vi "Top Level.vi"() -> ()   [LabVIEW 2020]
uses:
  Users/josferna/OneDrive - NI/Documents/Accounts&Proojects/Open Case Files/01072359 - Microsoft/rad-master/subVIs/rad_Globals.vi
  Users/josferna/OneDrive - NI/Documents/Accounts&Proojects/Open Case Files/01072359 - Microsoft/rad-master/subVIs/Util/Controls/Exit Button.ctl
  Users/josferna/OneDrive - NI/Documents/Accounts&Proojects/Open Case Files/01072359 - Microsoft/rad-master/subVIs/Util/FP Control/FP Control Functions.ctl
  <vilib>/Utility/miscctls.llb/LVRowAndColumnUnsignedTypeDef.ctl
  <vilib>/nisyscfg/nisyscfg.lvlib
  <resource>/objmgr/nisysapi.rc
  Users/josferna/OneDrive - NI/Documents/Accounts&Proojects/Open Case Files/01072359 - Microsoft/rad-master/subVIs/RT Image Compare/TypeDefs/rad_Comparison Modes.ctl
  Users/josferna/OneDrive - NI/Documents/Accounts&Proojects/Open Case Files/01072359 - Microsoft/rad-master/subVIs/Targets/TypeDefs/rad_Target Network Settings.ctl
  Users/josferna/OneDrive - NI/Documents/Accounts&Proojects/Open Case Files/01072359 - Microsoft/rad-master/subVIs/Targets/TypeDefs/rad_Target Information.ctl
  <vilib>/nisyscfg/Close (System).vi
  Users/josferna/OneDrive - NI/Documents/Accounts&Proojects/Open Case Files/01072359 - Microsoft/rad-master/subVIs/Util/Controls/Refresh Button.ctl
  Users/josferna/OneDrive - NI/Documents/Accounts&Proojects/Open Case Files/01072359 - Microsoft/rad-master/subVIs/Util/Controls/Add Target Button.ctl
  Users/josferna/OneDrive - NI/Documents/Accounts&Proojects/Open Case Files/01072359 - Microsoft/rad-master/subVIs/Util/Controls/Configure Button.ctl
  Users/josferna/OneDrive - NI/Documents/Accounts&Proojects/Open Case Files/01072359 - Microsoft/rad-master/subVIs/Util/Controls/Select All Button.ctl
  Users/josferna/OneDrive - NI/Documents/Accounts&Proojects/Open Case Files/01072359 - Microsoft/rad-master/subVIs/Util/Controls/Compare Button.ctl
  Users/josferna/OneDrive - NI/Documents/Accounts&Proojects/Open Case Files/01072359 - Microsoft/rad-master/subVIs/Util/Controls/Retrieve Button.ctl
  Users/josferna/OneDrive - NI/Documents/Accounts&Proojects/Open Case Files/01072359 - Microsoft/rad-master/subVIs/Util/Controls/Deploy Button.ctl
  Users/josferna/OneDrive - NI/Documents/Accounts&Proojects/Open Case Files/01072359 - Microsoft/rad-master/subVIs/App Images/TypeDefs/rad_FPGA Flash Properties.ctl
  Users/josferna/OneDrive - NI/Documents/Accounts&Proojects/Open Case Files/01072359 - Microsoft/rad-master/subVIs/App Images/TypeDefs/rad_FPGA Properties.ctl
  Users/josferna/OneDrive - NI/Documents/Accounts&Proojects/Open Case Files/01072359 - Microsoft/rad-master/subVIs/App Images/TypeDefs/rad_Application Image Properties.ctl
  Users/josferna/OneDrive - NI/Documents/Accounts&Proojects/Open Case Files/01072359 - Microsoft/rad-master/subVIs/App Images/TypeDefs/rad_AppImage Information.ctl
  Users/josferna/OneDrive - NI/Documents/Accounts&Proojects/Open Case Files/01072359 - Microsoft/rad-master/subVIs/App Images/TypeDefs/rad_App Images Settings.ctl
  Users/josferna/OneDrive - NI/Documents/Accounts&Proojects/Open Case Files/01072359 - Microsoft/rad-master/subVIs/Targets/TypeDefs/rad_Targets Settings.ctl
  Users/josferna/OneDrive - NI/Documents/Accounts&Proojects/Open Case Files/01072359 - Microsoft/rad-master/subVIs/Targets/TypeDefs/rad_Discovery Settings.ctl
  Users/josferna/OneDrive - NI/Documents/Accounts&Proojects/Open Case Files/01072359 - Microsoft/rad-master/subVIs/TypeDefs/rad_State Data.ctl
panel:
  in  "App Images List 2":i32(listbox)=6
  in  "Target List 2":i32[](listbox)=[0]
  in  "State":T1 {"Targets Information"."Primary NIC"."IP Address Request Mode" items=["Static"=1, "DHCP/Link-Local"=2, "Link-Local Only"=4, "DHCP Only"=8]}
  in  "Exit":T11
  in  "Deploy":T12
  in  "Retrieve":T13
  in  "Compare":T14
  in  "Configure App":T15
  in  "Select All":T16
  in  "Configure Targets":T15
  in  "App Images Settings":bool
  in  "Add Target":T17
  in  "Targets Settings":bool
  in  "Refresh Apps":T18
  in  "App Images List":i32(listbox)=6
  in  "Target List":i32[](listbox)=[0]
  in  "Refresh Targets":T18
  # "Deployment Targets"
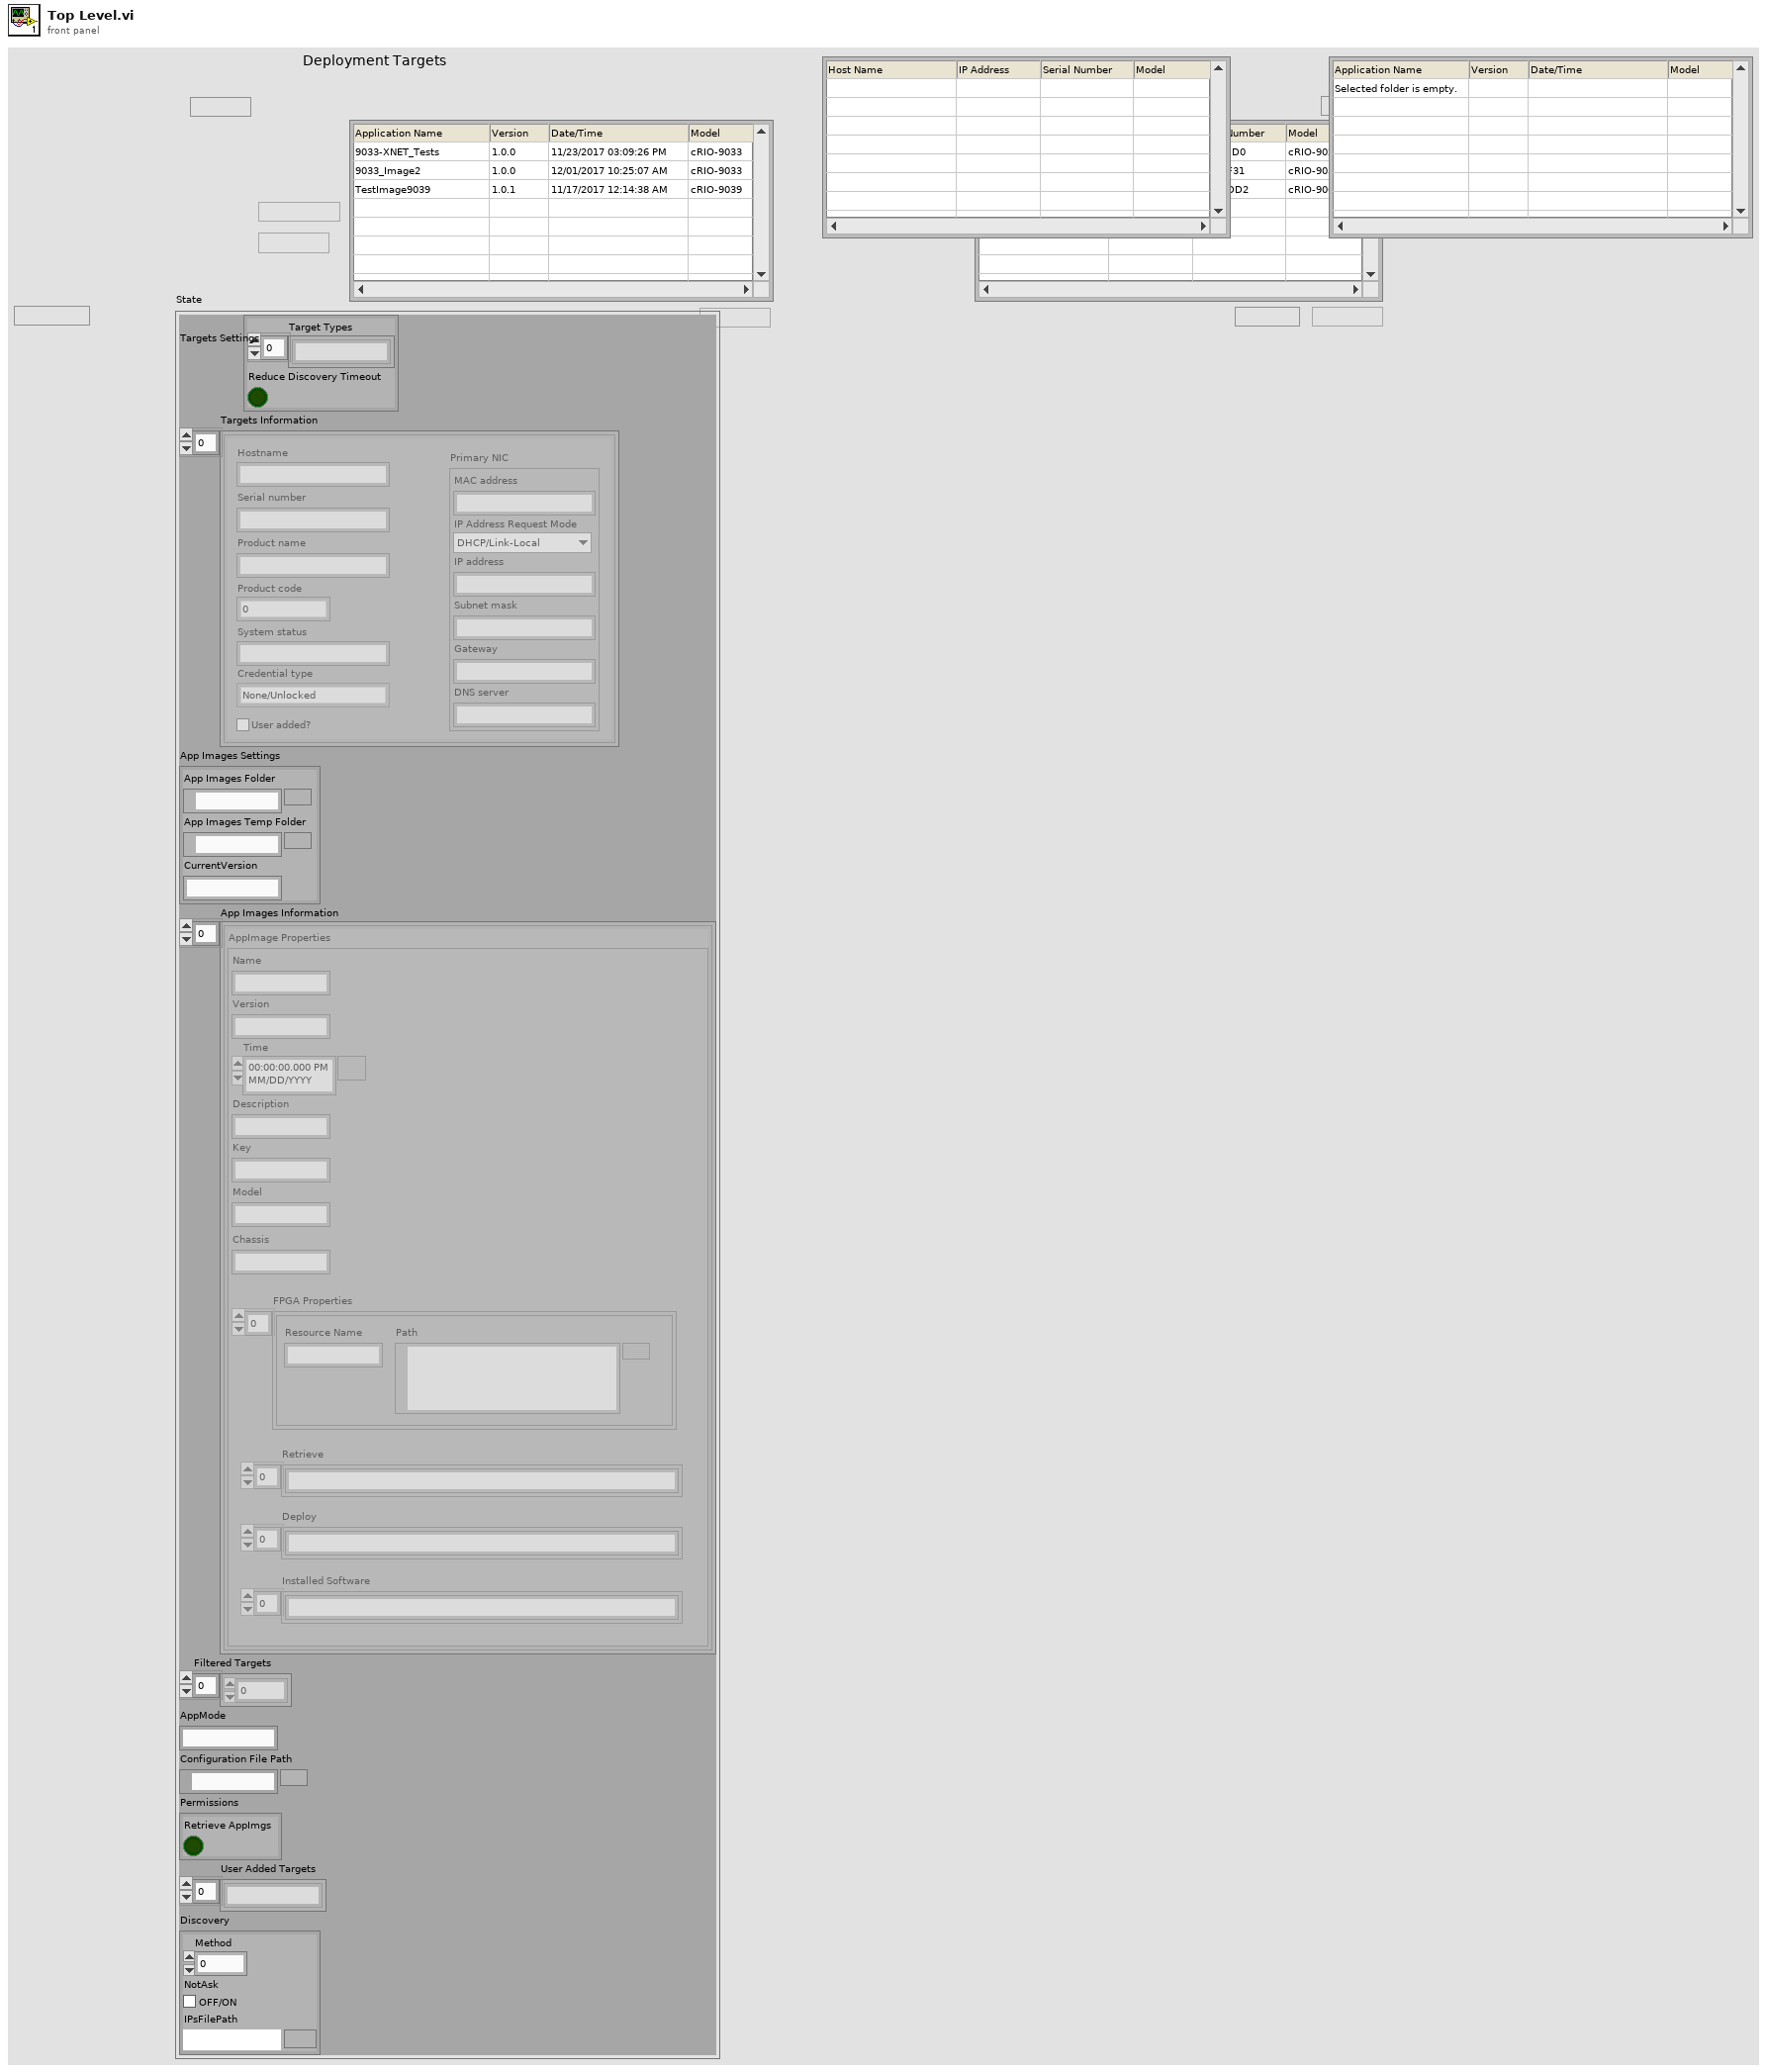
[diagram p1: front panel]
types:
  T1 = typedef "rad_State Data.ctl" = cluster{"Targets Settings":T2, "Targets Information":T3[], "App Images Settings":T5, "App Images Information":T6[], "Filtered Targets":i32[], "AppMode":string, "Configuration File Path":path, "Permissions":cluster{"Retrieve AppImgs":bool}, "User Added Targets":string[], "Discovery":T10}
  T2 = typedef "rad_Targets Settings.ctl" = cluster{"Target Types":string[], "Reduce Discovery Timeout":bool}
  T3 = typedef "rad_Target Information.ctl" = cluster{"Hostname":string, "Serial number":string, "Product name":string, "Product code":i32, "System status":string, "Credential type":enum16{"None/Unlocked", "FTP Password", "NIAuth Credentials"}, "User added?":bool, "Primary NIC":T4}
  T4 = typedef "rad_Target Network Settings.ctl" = cluster{"MAC address":string, "IP Address Request Mode":i32, "IP address":string, "Subnet mask":string, "Gateway":string, "DNS server":string}
  T5 = typedef "rad_App Images Settings.ctl" = cluster{"App Images Folder":path, "App Images Temp Folder":path, "CurrentVersion":string}
  T6 = typedef "rad_AppImage Information.ctl" = cluster{"AppImage Properties":T7, "AppImage Path":path}
  T7 = typedef "rad_Application Image Properties.ctl" = cluster{"Name":string, "Version":string, "Time":timestamp, "Description":string, "Key":string, "Chassis":string, "FPGA Properties":T8, "Model":string, "Retrieve":string[], "Deploy":string[], "Installed Software":string[]}
  T8 = typedef "rad_FPGA Properties.ctl" = T9[]
  T9 = typedef "rad_FPGA Flash Properties.ctl" = cluster{"Resource Name":string, "Path":path}
  T10 = typedef "rad_Discovery Settings.ctl" = cluster{"Method":u32, "NotAsk":bool, "IPsFilePath":path}
  T11 = typedef "Exit Button.ctl" = bool
  T12 = typedef "Deploy Button.ctl" = bool
  T13 = typedef "Retrieve Button.ctl" = bool
  T14 = typedef "Compare Button.ctl" = bool
  T15 = typedef "Configure Button.ctl" = bool
  T16 = typedef "Select All Button.ctl" = bool
  T17 = typedef "Add Target Button.ctl" = bool
  T18 = typedef "Refresh Button.ctl" = bool
  T19 = typedef "LVPoint32TypeDef.ctl" = cluster{"Horizontal":i32, "Vertical":i32}
  T20 = typedef "LVRowAndColumnTypeDef.ctl" = cluster{"Row":i32, "Column":i32}
  T21 = typedef "FP Control Functions.ctl" = enum16{"Open", "Close", "Bring To Front", "Center"}
  T22 = typedef "LVRowAndColumnUnsignedTypeDef.ctl" = cluster{"Row":u32, "Column":u32}
  T23 = typedef "rad_Comparison Modes.ctl" = enum32{"Compare Local Image With Controller", "Compare Two Local Images"}
  T24 = enum8{"Enabled", "Disabled", "Disabled and Grayed Out"}
  T25 = enum32{"invalid app kind", "Development System", "Run Time System", "Student Edition", "Embedded LabVIEW", "Evaluation", "Custom"}
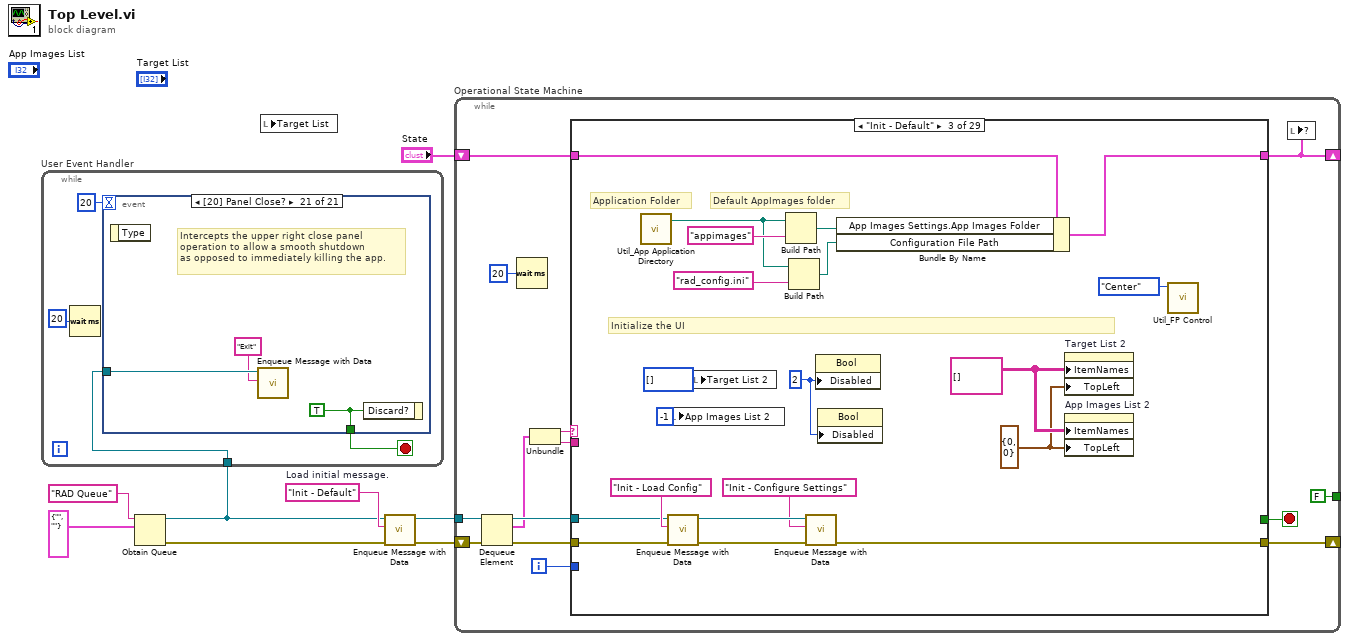
[diagram p0: block diagram]
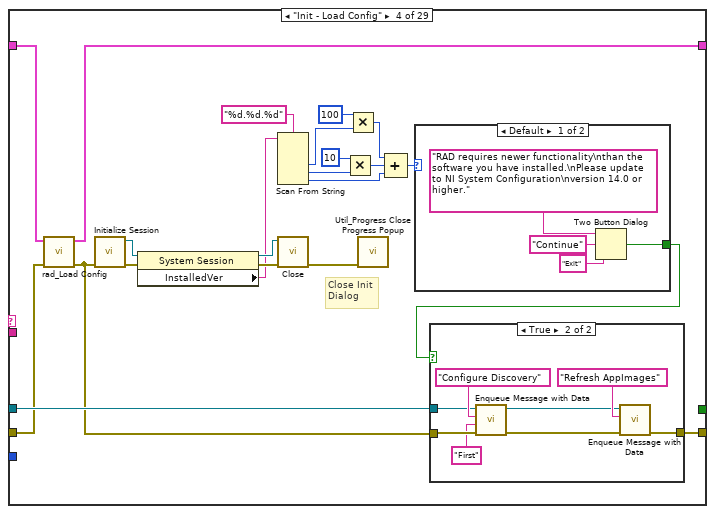
[diagram p4: hidden frame]
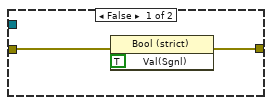
[diagram p5: hidden frame]
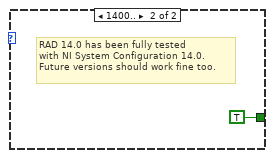
[diagram p6: hidden frame]
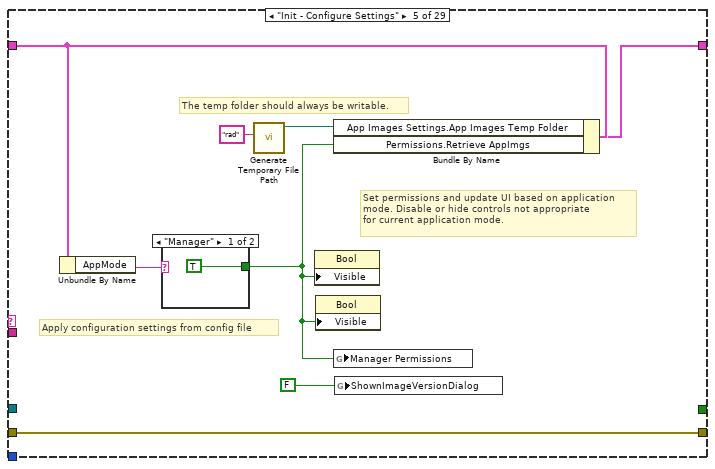
[diagram p7: hidden frame]
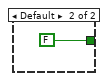
[diagram p8: hidden frame]
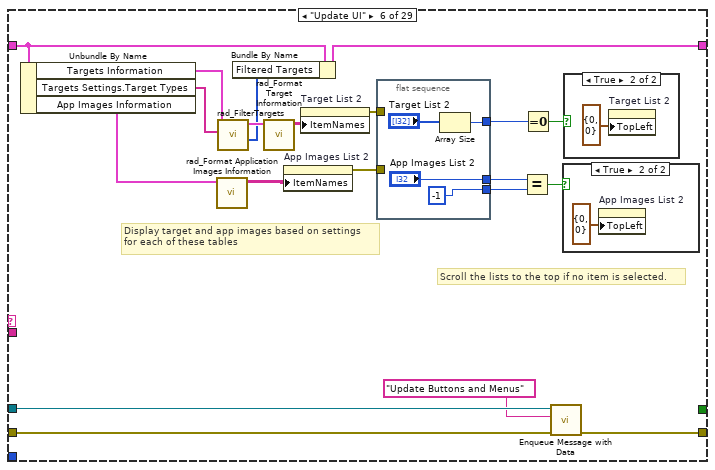
[diagram p9: hidden frame]
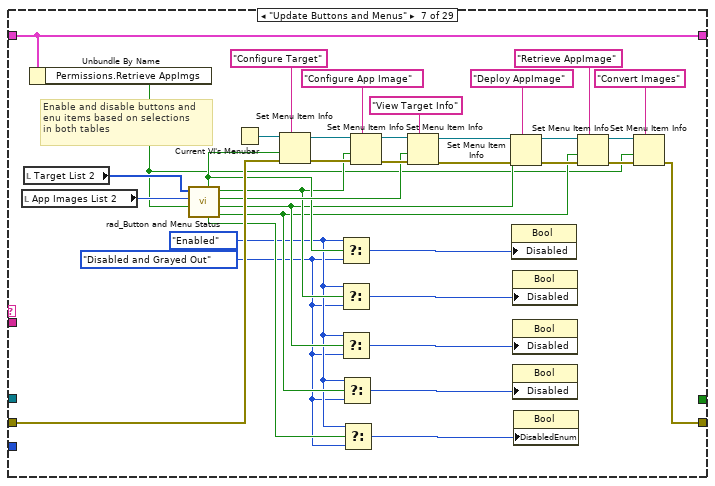
[diagram p12: hidden frame]
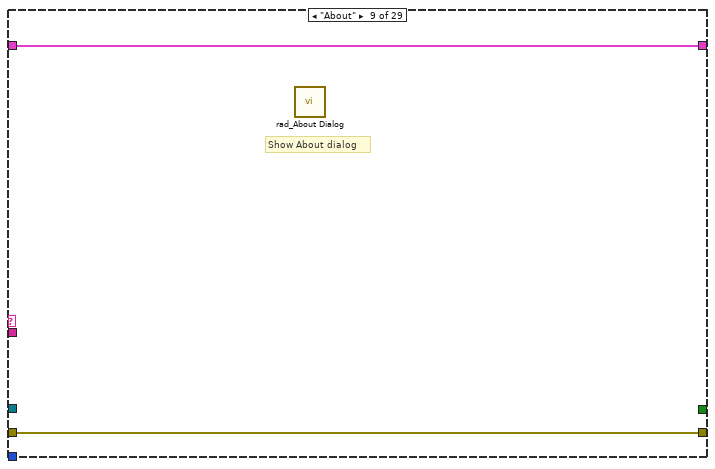
[diagram p14: hidden frame]
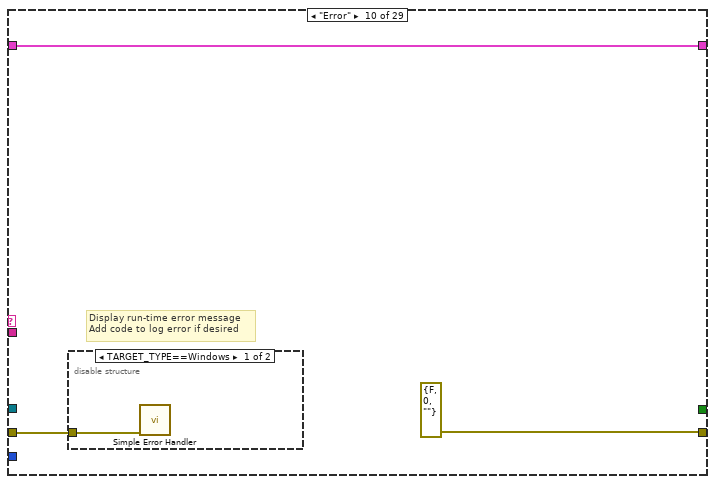
[diagram p15: hidden frame]
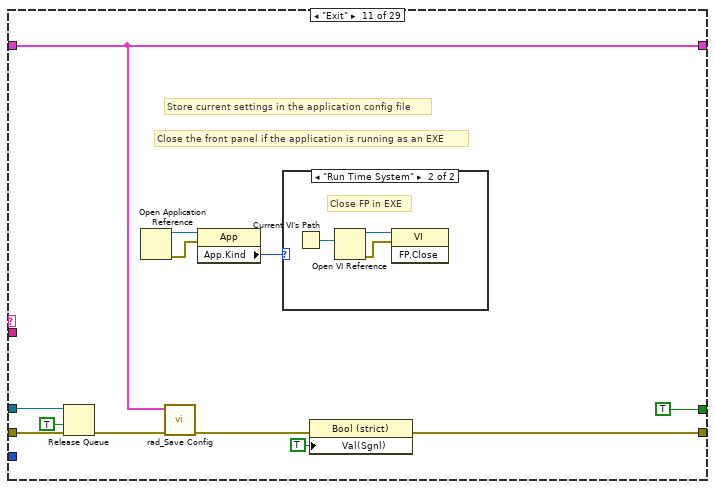
[diagram p17: hidden frame]
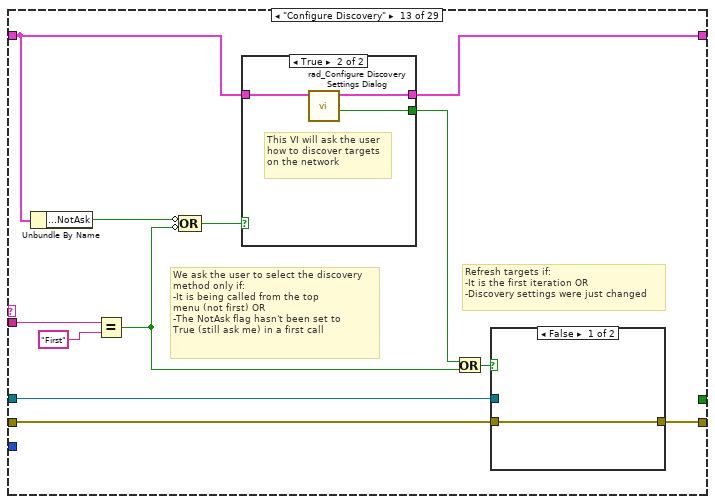
[diagram p20: hidden frame]
diagram:
  w5 = "Init - Default"  # Load initial message.
  n1 = Obtain Queue(name (unnamed)="RAD Queue" ("message queue name"), element data type=cluster{string, string} {"", ""}) -> (queue out=w2:refnum<queue>, error out=w1:errorcluster)  [unwired: 3 in, 1 out]
  n2 = while "User Event Handler" {
    tunnel: w2 -> [w10]
    stop <- w11 stop-if-true
    n3 = Wait (ms)(milliseconds to wait=u32 20) -> ()  [unwired: 1 out]
    n4 = event shown="[20] Panel Close?" {
      selector: _ -> [_ _ _ _ _ _ _ _ _ _ _ _ _ _ _ _ _ _ _ _ _]
      dyn-events: _ -> [_ _ _ _ _ _ _ _ _ _ _ _ _ _ _ _ _ _ _ _ _]
      timeout: 20 -> [_ _ _ _ _ _ _ _ _ _ _ _ _ _ _ _ _ _ _ _ _]
      tunnel: [w17 _ _ _ _ _ _ _ _ _ _ _ _ _ _ _ _ _ _ TRUE ("Discard?") w137] -> w11
      tunnel: w10 -> [w19 w21 w23 w25 w27 w29 w33 _ w42 _ w53 w55 w59 w73 w77 w90 w108 _ w127 w133 w136]
      event Timeout {
        # "Check status of message queue on Timeout\nStop loop if message queue has been destroyed"
        n5 = event-data() -> ()  [unwired: 2 out]
        n6 = control-ref of="This VI"() -> (w13:refnum<vi>)
        n7 = property class="VI"(reference=w13) -> (error out=w14:errorcluster, "Panel"=w16:refnum<vi>)  [unwired: 1 in, 1 out]
        n8 = Get Queue Status(queue=w19) -> (error out=w18:errorcluster)  [unwired: 1 in, 8 out]
        n9 = property class="Pnl"(reference=w16, error in=w14, "DeferPanUpdts"=FALSE ("Defer Panel Updates")) -> ()  [unwired: 2 out]
        n10 = Unbundle By Name(w18) -> ("status"=w17:bool)
      }
      event Value Change {
        n11 = event-data() -> ()  [unwired: 2 out]
        n12 = call "Enqueue Message with Data.vi"("message ID"="Refresh Targets", "queue in"=w21) -> ()  [unwired: 8 in, 2 out]
      }
      event Value Change {
        n13 = event-data() -> ()  [unwired: 2 out]
        n14 = call "Enqueue Message with Data.vi"("message ID"="Refresh AppImages", "queue in"=w23) -> ()  [unwired: 8 in, 2 out]
      }
      event "Targets Settings": Value Change {
        # "UNUSE"
        n15 = event-data() -> ()  [unwired: 2 out]
        n16 = call "Enqueue Message with Data.vi"("message ID"="Configure Targets Settings", "queue in"=w25) -> ()  [unwired: 8 in, 2 out]
      }
      event Value Change {
        # "UNUSED"
        n17 = event-data() -> ()  [unwired: 2 out]
        n18 = call "Enqueue Message with Data.vi"("message ID"="Add Target to List" ("Message Name"), "queue in"=w27) -> ()  [unwired: 8 in, 2 out]
      }
      event "App Images Settings": Value Change {
        n19 = event-data() -> ()  [unwired: 2 out]
        n20 = call "Enqueue Message with Data.vi"("message ID"="Configure AppImages Settings", "queue in"=w29) -> ()  [unwired: 8 in, 2 out]
      }
      event Value Change {
        n21 = event-data() -> ()  [unwired: 2 out]
        n22 = local read "Target List"() -> (w30:i32[])
        n23 = Index Array(array=w30) -> (element=w34:i32)  [unwired: 1 in]
        n24 = Number To Decimal String(number=w34) -> (decimal integer string=w31:string)  [unwired: 1 out]
        n25 = call "Enqueue Message with Data.vi"("extra data"=w31, "message ID"="Configure Target", "queue in"=w33) -> ()  [unwired: 7 in, 2 out]
      }
      event Value Change {
        n26 = event-data() -> ()  [unwired: 2 out]
        n27 = local read "State"() -> (w38:T1)
        n28 = Unbundle By Name(w38) -> ("Targets Information"=w37:T3[])
        n29 = Array Size(array=w37) -> (size(s)=w36:i32)
        n30 = for {
          N: w36 -> [_]
          tunnel: [w39] -> w35 mode=indexing
          i -> [w39]
        }
        n31 = local write "Target List"(w35) -> ()
      }
      event Value Change {
        # "UNUSED"
        n32 = event-data() -> ()  [unwired: 2 out]
        n33 = local read "App Images List"() -> (w43:i32)
        n34 = Number To Decimal String(number=w43) -> (decimal integer string=w40:string)  [unwired: 1 out]
        n35 = call "Enqueue Message with Data.vi"("extra data"=w40, "message ID"="Configure App Image", "queue in"=w42) -> ()  [unwired: 7 in, 2 out]
      }
      event "App Images List": Mouse Down? {
        w47 = 0 ("index (row)")
        # "Discard a selection if the image list is empty."
        n36 = event-data() -> ("CtlRef"=w49:refnum<vi>)  [unwired: 1 out]
        n37 = global read "rad_Globals.vi" "Empty List Message"() -> (w45:string)
        n38 = property class="MCListbox (strict)"(reference=w49) -> ("ItemNames"=w48:string[][])  [unwired: 1 in, 2 out]
        n39 = Index Array(array=w48, index (row)=w47, index (col)=w47) -> (element=w46:string)
        n40 = Equal?(x=w46, y=w45) -> (x = y?=w44:bool)
        n41 = event-data("Discard?"=w44) -> ()  [unwired: 1 in, 1 out]
      }
      event "Target List": Value Change {
        n42 = event-data() -> ("CtlRef"=w51:refnum<vi>)  [unwired: 1 out]
        n43 = call "rad_Filter Disconnected Targets.vi"("Target List Ref"=w51) -> ("error out"=w50:errorcluster)  [unwired: 10 in]
        n44 = call "Enqueue Message with Data.vi"("error in (no error)"=w50, "message ID"="Update UI" ("Message"), "queue in"=w53) -> ()  [unwired: 7 in, 2 out]
      }
      event "App Images List": Value Change {
        n45 = event-data() -> ()  [unwired: 2 out]
        n46 = call "Enqueue Message with Data.vi"("message ID"="Update UI" ("Message"), "queue in"=w55) -> ()  [unwired: 8 in, 2 out]
      }
      event Value Change {
        # "UNUSED"
        # "Message Value example: (1,2,7,):0"
        n47 = event-data() -> ()  [unwired: 2 out]
        n48 = local read "Target List"() -> (w56:i32[])
        n49 = local read "App Images List"() -> (w62:i32)
        n50 = for {
          shift-right: [w69] -> w63
          shift-left: "(" -> [w67]
          tunnel: w56 -> [w68] mode=indexing
          n51 = Format Into String(format string="%d,", initial string=w67, w68) -> (resulting string=w69:string)  [unwired: 1 in, 1 out]
        }
        n52 = Number To Decimal String(number=w62) -> (decimal integer string=w61:string)  [unwired: 1 out]
        n53 = Concatenate Strings("Image Target Compare" ("string"), w63, "):" ("string"), w61) -> (w65:string)
        n54 = call "Enqueue Message with Data.vi"("extra data"=w65, "message ID"="Compare App Image", "queue in"=w59) -> ()  [unwired: 7 in, 2 out]
      }
      event Value Change {
        # "UNUSED"
        n55 = event-data() -> ()  [unwired: 2 out]
        n56 = local read "Target List"() -> (w70:i32[])
        n57 = Index Array(array=w70) -> (element=w74:i32)  [unwired: 1 in]
        n58 = Number To Decimal String(number=w74) -> (decimal integer string=w71:string)  [unwired: 1 out]
        n59 = call "Enqueue Message with Data.vi"("extra data"=w71, "message ID"="Retrieve AppImage", "queue in"=w73) -> ()  [unwired: 7 in, 2 out]
      }
      event Value Change {
        # "Request to deploy app imaghe to multiple targets"
        # "Message Value example: (1,2,7,):0"
        n60 = event-data() -> ()  [unwired: 2 out]
        n61 = local read "Target List"() -> (w79:i32[])
        n62 = local read "App Images List"() -> (w81:i32)
        n63 = for {
          shift-right: [w87] -> w78
          shift-left: "(" -> [w85]
          tunnel: w79 -> [w86] mode=indexing
          n64 = Format Into String(format string="%d,", initial string=w85, w86) -> (resulting string=w87:string)  [unwired: 1 in, 1 out]
        }
        n65 = Number To Decimal String(number=w81) -> (decimal integer string=w82:string)  [unwired: 1 out]
        n66 = Concatenate Strings(w78, "):" ("string"), w82) -> (w75:string)
        n67 = call "Enqueue Message with Data.vi"("extra data"=w75, "message ID"="Deploy AppImage", "queue in"=w77) -> ()  [unwired: 7 in, 2 out]
      }
      event Menu Selection (User) {
        # "EDIT MENU"
        # "Process menu interactions"
        n68 = event-data() -> ("ItemTag"=w91:string)  [unwired: 1 out]
        n69 = case shown="\"Configure Target\"" w91 {
          selector: w91 -> [w92 w94 w98 w102 w104]
          tunnel: [w92 w94 w98 w102 w104] -> w89
          tunnel: [_ w93 w97 w101 "Generic Compare"] -> w88
          frame Default {
          }
          frame "Configure Target" {
            n70 = local read "Target List"() -> (w96:i32[])
            n71 = Index Array(array=w96) -> (element=w95:i32)  [unwired: 1 in]
            n72 = Number To Decimal String(number=w95) -> (decimal integer string=w93:string)  [unwired: 1 out]
          }
          frame "View Target Info" {
            n73 = local read item#-1() -> (w100)
            n74 = Index Array(array=w100) -> (element=w99)  [unwired: 1 in]
            n75 = Number To Decimal String(number=w99) -> (decimal integer string=w97:string)  [unwired: 1 out]
          }
          frame "Configure App Image" {
            n76 = local read "App Images List"() -> (w103:i32)
            n77 = Number To Decimal String(number=w103) -> (decimal integer string=w101:string)  [unwired: 1 out]
          }
          frame "Compare App Image" {
          }
        }
        n78 = call "Enqueue Message with Data.vi"("extra data"=w88, "message ID"=w89, "queue in"=w90) -> ()  [unwired: 7 in, 2 out]
      }
      event "Target List": Shortcut Menu Selection (User) {
        n79 = event-data() -> ("CtlRef"=w110:refnum<vi>, "Coords"=w109:T19, "ItemTag"=w107:string)  [unwired: 2 out]
        n80 = invoke class="MCListbox (strict)" method="Point To Row Column"(reference=w110, "Point"=w109) -> ("CellPosition"=w112:T20)  [unwired: 5 in, 6 out]
        n81 = Unbundle By Name(w112) -> ("Row"=w111:i32)
        n82 = Number To Decimal String(number=w111) -> (decimal integer string=w106:string)  [unwired: 1 out]
        n83 = call "Enqueue Message with Data.vi"("extra data"=w106, "message ID"=w107, "queue in"=w108) -> ()  [unwired: 7 in, 2 out]
      }
      event "App Images List": Shortcut Menu Activation? {
        n84 = event-data() -> ("MenuRef"=w114:refnum<k9>)  [unwired: 1 out]
        n85 = global read "rad_Globals.vi" "Manager Permissions"() -> (w113:bool)
        n86 = case shown="False" w113 {
          tunnel: w114 -> [w119 _]
          tunnel: [w116 _] -> _
          frame False {
            w115 = string[] ["View App Image Info"] ("item names")
            n87 = Delete Menu Items(9:w119) -> (0:w117:errorcluster, 3:w118:refnum<k9>)  [unwired: 3 in]
            n88 = Insert Menu Items(6:w117, 7:w115, 8:w115, 9:w118) -> (0:w116:errorcluster)  [unwired: 2 in, 2 out]
          }
          frame True {
          }
        }
        n89 = event-data() -> ()  [unwired: 2 in, 1 out]
      }
      event "App Images List": Shortcut Menu Selection (User) {
        n90 = event-data() -> ("CtlRef"=w129:refnum<vi>, "Coords"=w128:T19, "ItemTag"=w120:string)  [unwired: 1 out]
        n91 = Equal?(x=w120, y="Compare App Image") -> (x = y?=w125:bool)
        n92 = invoke class="MCListbox (strict)" method="Point To Row Column"(reference=w129, "Point"=w128) -> ("CellPosition"=w131:T20)  [unwired: 5 in, 6 out]
        n93 = Unbundle By Name(w131) -> ("Row"=w130:i32)
        n94 = Number To Decimal String(number=w130) -> (decimal integer string=w122:string)  [unwired: 1 out]
        n95 = Concatenate Strings("Only Image Selected(" ("string"), w122) -> (w124:string)
        n96 = Select(t=w124, s=w125, f=w122) -> (s? t:f=w121:string)
        n97 = call "Enqueue Message with Data.vi"("extra data"=w121, "message ID"=w120, "queue in"=w127) -> ()  [unwired: 7 in, 2 out]
      }
      event Value Change {
        n98 = event-data() -> ()  [unwired: 2 out]
        n99 = call "Enqueue Message with Data.vi"("message ID"="Exit", "queue in"=w133) -> ()  [unwired: 8 in, 2 out]
      }
      event Panel Close? {
        w137 = TRUE ("Discard?")
        # "Intercepts the upper right close panel\noperation to allow a smooth shutdown\nas opposed to immediately killing the app."
        n100 = event-data() -> ()  [unwired: 2 out]
        n101 = call "Enqueue Message with Data.vi"("message ID"="Exit", "queue in"=w136) -> ()  [unwired: 8 in, 2 out]
        n102 = event-data("Discard?"=w137) -> ()  [unwired: 1 in, 1 out]
      }
    }
  }
  n103 = local read "Target List"() -> ()  [unwired: 1 in]
  n104 = call "Enqueue Message with Data.vi"("error in (no error)"=w1, "message ID"=w5, "queue in"=w2) -> ("error out"=w3:errorcluster, "queue out"=w4:refnum<queue>)  [unwired: 7 in]
  n105 = while "Operational State Machine" {
    shift-left: w3 -> [w143]
    shift-right: [w144] -> _
    tunnel: w4 -> [w148]
    shift-left: "State" -> [w151]
    shift-right: [w145] -> _
    tunnel: [T11 FALSE ("Exit")] -> _
    i -> [w147]
    stop <- w141 stop-if-true
    n106 = Dequeue Element(queue=w148, error in (no error)=w143) -> (queue out=w150:refnum<queue>, element=w146:cluster{string, string}, error out=w149:errorcluster)  [unwired: 1 in, 1 out]
    n107 = Wait (ms)(milliseconds to wait=u32 20) -> ()  [unwired: 1 out]
    n108 = Unbundle(w146) -> (w140:string, w139:string)
    n109 = case shown="\"Init - Default\"" w140 {
      tunnel: [w153 w155 w169 w197 w219 w240 w271 w286 w288 w292 w298 w310 w322 w340 w356 w378 w394 w410 w423 w434 w436 w457 w472 w484 w492 w561 w576 w608 w624] -> w145
      tunnel: w151 -> [w153 w155 w173 w196 w220 w236 w271 w286 w288 w292 w298 w310 w316 w341 w357 w379 w395 w410 w428 w434 w440 w458 w471 w484 w492 w561 w577 w608 w624]
      tunnel: w150 -> [_ _ w157 w180 _ w232 _ _ _ _ w305 _ w320 w338 w352 w377 w393 _ w422 _ w438 w451 w474 _ _ w548 w580 w593 w625]
      tunnel: w149 -> [w152 w154 w162 w179 w218 w234 w268 w287 w289 w291 w304 w309 w319 w337 w354 w373 w392 w403 w421 w433 w437 w453 w473 w485 w491 w550 w583 w596 w629]
      tunnel: w147 -> [_ _ _ _ _ _ _ _ _ _ _ _ _ _ _ _ _ _ _ _ _ _ _ _ _ _ _ _ _]
      tunnel: w139 -> [_ _ _ _ _ _ _ _ _ _ _ _ w313 _ _ w387 _ w408 w432 _ _ w461 _ w481 w488 w559 w585 w607 _]
      tunnel: [w152 w154 w156 w181 w218 w233 w252 w287 w289 errorcluster {"status"=FALSE, "code"=0, "source"=""} ("error out") w299 w309 w321 w339 w353 w375 w389 w403 w420 w433 w439 w452 w468 w485 w486 w549 w581 w595 w626] -> w144
      tunnel: [_ _ _ _ _ _ _ _ _ _ TRUE _ _ _ _ _ _ _ _ _ _ _ _ _ _ _ _ _ _] -> w141
      frame "Missing Message Handler", Default {
      }
      frame "**** General Application Messages ****" {
      }
      frame "Init - Default" {
        w163 = T22 {"Row"=0, "Column"=0} ("Top Left Visible Cell")
        w165 = string[][] [] ("Item Names")
        w172 = u8 2 ("Disabled")
        # "Initialize the UI"
        # "Application Folder"
        # "Default AppImages folder"
        n110 = call "Util_App Application Directory.vi"() -> ("Application Directory"=w168:path)  [unwired: 11 out]
        n111 = call "Enqueue Message with Data.vi"("error in (no error)"=w162, "message ID"="Init - Load Config", "queue in"=w157) -> ("error out"=w161:errorcluster, "queue out"=w160:refnum<queue>)  [unwired: 7 in]
        n112 = local write "App Images List 2"(-1 ("App Images List")) -> ()
        n113 = local write "Target List 2"(i32[] [] ("Target List")) -> ()
        n114 = Build Path(base path=w168, name or relative path="appimages") -> (appended path=w174:path)
        n115 = Build Path(base path=w168, name or relative path="rad_config.ini" ("Config File Name")) -> (appended path=w166:path)
        n116 = call "Enqueue Message with Data.vi"("error in (no error)"=w161, "message ID"="Init - Configure Settings", "queue in"=w160) -> ("error out"=w156:errorcluster)  [unwired: 7 in, 1 out]
        n117 = property on="Property Node" class="Bool"("Disabled"=w172) -> ()  [unwired: 2 in, 2 out]
        n118 = property on="Property Node" class="Bool"("Disabled"=w172) -> ()  [unwired: 2 in, 2 out]
        n119 = Bundle By Name(cluster=w173, "App Images Settings.App Images Folder"=w174, "Configuration File Path"=w166) -> (w169:T1)
        n120 = property on="Target List 2" class="MCListbox (strict)"("ItemNames"=w165, "TopLeft"=w163) -> ()  [unwired: 2 in, 2 out]
        n121 = property on="App Images List 2" class="MCListbox (strict)"("ItemNames"=w165, "TopLeft"=w163) -> ()  [unwired: 2 in, 2 out]
        n122 = call "Util_FP Control.vi"("Function"=FP_Control_Functions."Center") -> ()  [unwired: 10 in, 1 out]
      }
      frame "Init - Load Config" {
        # "Close Init\nDialog"
        n123 = call "rad_Load Config.vi"("error in (no error"=w179, "State in"=w196) -> ("error out"=w177:errorcluster, "State out"=w197:T1)  [unwired: 1 in, 7 out]
        n124 = call <vilib>:"Initialize Session.vi"("error in (no error)"=w177) -> ("error out"=w184:errorcluster, "Session out"=w185:refnum<k21>)  [unwired: 9 in]
        n125 = property class="System Session"(reference=w185, error in=w184) -> (reference out=w186:refnum<k21>, error out=w183:errorcluster, "InstalledVer"=w182:string)
        n126 = Scan From String(format string="%d.%d.%d", input string=w182) -> (output 1=w194:i32, output 2=w191:i32, output 3=w188:i32)  [unwired: 5 in, 3 out]
        n127 = call-poly <vilib>:"Close.vi"("error in (no error)"=w183, "Session in"=w186) -> ("error out"=w176:errorcluster)  [unwired: 9 in]
        n128 = Multiply(x=10, y=w191) -> (x*y=w189:i32)
        n129 = Multiply(x=100, y=w194) -> (x*y=w190:i32)
        n130 = call "Util_Progress Close Progress Popup.vi"("error in (no error)"=w176) -> ()  [unwired: 2 in, 9 out]
        n131 = Compound Arithmetic op=ADD(w190, w189, w188) -> (w187:i32)
        n132 = case shown="Default" w187 {
          tunnel: [w209 TRUE ("T button?")] -> w178
          frame Default {
            n133 = Two Button Dialog(message="RAD requires newer functionality\nthan the software you have installed.\nPlease update to NI System Configuration\nversion 14.0 or higher.", 1:"Exit" ("F button name (\"Cancel\")"), 2:"Continue" ("T button name (\"OK\")")) -> (T button?=w209:bool)
          }
          frame 1400.. {
            # "RAD 14.0 has been fully tested\nwith NI System Configuration 14.0.\nFuture versions should work fine too."
          }
        }
        n134 = case shown="True" w178 {
          tunnel: w177 -> [w199 w207]
          tunnel: [w200 w202] -> w181
          tunnel: w180 -> [_ w206]
          frame False {
            n135 = property on="Property Node" class="Bool (strict)"(error in=w199, "Val(Sgnl)"=T11 TRUE ("Value (Signaling)")) -> (error out=w200:errorcluster)  [unwired: 1 in, 1 out]
          }
          frame True {
            n136 = call "Enqueue Message with Data.vi"("error in (no error)"=w207, "extra data"="First", "message ID"="Configure Discovery", "queue in"=w206) -> ("error out"=w203:errorcluster, "queue out"=w204:refnum<queue>)  [unwired: 6 in]
            n137 = call "Enqueue Message with Data.vi"("error in (no error)"=w203, "message ID"="Refresh AppImages", "queue in"=w204) -> ("error out"=w202:errorcluster)  [unwired: 7 in, 1 out]
          }
        }
      }
      frame "Init - Configure Settings" {
        # "The temp folder should always be writable."
        # "Set permissions and update UI based on application\nmode. Disable or hide controls not appropriate\nfor current application mode."
        # "Apply configuration settings from config file"
        n138 = Unbundle By Name(w220) -> ("AppMode"=w221:string)
        n139 = case shown="\"Manager\"" w221 {
          tunnel: [TRUE ("Visible") FALSE ("Visible")] -> w217
          frame "Manager" {
          }
          frame Default {
          }
        }
        n140 = call <vilib>:"Generate Temporary File Path.vi"("Temporary File Extension (tmp)"="rad") -> ("Unique Temporary File Path"=w214:path)  [unwired: 9 in, 1 out]
        n141 = property on="Property Node" class="Bool"("Visible"=w217) -> ()  [unwired: 2 in, 2 out]
        n142 = property on="Property Node" class="Bool"("Visible"=w217) -> ()  [unwired: 2 in, 2 out]
        n143 = Bundle By Name(cluster=w220, "App Images Settings.App Images Temp Folder"=w214, "Permissions.Retrieve AppImgs"=w217) -> (w219:T1)
        n144 = global write "rad_Globals.vi" "Manager Permissions"(w217) -> ()
        n145 = global write "rad_Globals.vi" "ShownImageVersionDialog"(FALSE ("ShownNewerVersionDialog")) -> ()
      }
      frame "Update UI" {
        # "Scroll the lists to the top if no item is selected."
        # "Display target and app images based on settings\nfor each of these tables"
        n146 = Unbundle By Name(w236) -> ("Targets Information"=w243:T3[], "Targets Settings.Target Types"=w235:string[], "App Images Information"=w237:T6[])
        n147 = call "rad_Format Application Images Information.vi"("App Images Information"=w237) -> ("App Images Information"=w238:string[][])  [unwired: 10 out]
        n148 = call "rad_FilterTargets.vi"("Target Types"=w235, "Targets Information"=w243) -> ("Filtered Targets"=w241:i32[], "Targets Information"=w242:T3[])  [unwired: 8 out]
        n149 = Bundle By Name(cluster=w236, "Filtered Targets"=w241) -> (w240:T1)
        n150 = call "rad_Format Target Information.vi"("Targets Information"=w242) -> ("Targets Information"=w239:string[][])  [unwired: 10 out]
        n151 = property on="App Images List 2" class="MCListbox (strict)"("ItemNames"=w238) -> (error out=w229:errorcluster)  [unwired: 2 in, 1 out]
        n152 = property on="Target List 2" class="MCListbox (strict)"("ItemNames"=w239) -> (error out=w230:errorcluster)  [unwired: 2 in, 1 out]
        n153 = flat-sequence {
          tunnel: w230 -> [_]
          tunnel: w229 -> [_]
          tunnel: ["App Images List 2"] -> w227
          tunnel: [w247] -> w228
          tunnel: [-1 ("y")] -> w225
          frame #0 {
            n154 = Array Size(array="Target List 2") -> (size(s)=w247:i32)
          }
        }
        n155 = Equal?(x=w227, y=w225) -> (x = y?=w224:bool)
        n156 = Equal To 0?(x=w228) -> (x = 0?=w226:bool)
        n157 = call "Enqueue Message with Data.vi"("error in (no error)"=w234, "message ID"="Update Buttons and Menus" ("Message Name"), "queue in"=w232) -> ("error out"=w233:errorcluster)  [unwired: 7 in, 1 out]
        n158 = case shown="True" w224 {
          frame False {
          }
          frame True {
            n159 = property on="App Images List 2" class="MCListbox (strict)"("TopLeft"=T22 {"Row"=0, "Column"=0} ("Top Left Visible Cell")) -> ()  [unwired: 2 in, 2 out]
          }
        }
        n160 = case shown="True" w226 {
          frame False {
          }
          frame True {
            n161 = property on="Target List 2" class="MCListbox (strict)"("TopLeft"=T22 {"Row"=0, "Column"=0} ("Top Left Visible Cell")) -> ()  [unwired: 2 in, 2 out]
          }
        }
      }
      frame "Update Buttons and Menus" {
        w256 = T24."Disabled and Grayed Out" ("Disabled")
        w257 = T24."Enabled" ("Disabled")
        # "Enable and disable buttons and \nenu items based on selections\nin both tables"
        n162 = local read "App Images List 2"() -> (w269:i32)
        n163 = local read "Target List 2"() -> (w270:i32[])
        n164 = Unbundle By Name(w271) -> ("Permissions.Retrieve AppImgs"=w250:bool)
        n165 = call "rad_Button and Menu Status.vi"("Manager Permissions"=w250, "App Image List"=w269, "Target List"=w270) -> ("Retrieve AppImage"=w260:bool, "Deploy AppImage"=w262:bool, "View Target Info"=w267:bool, "Configure App Image"=w264:bool, "Compare"=w258:bool, "Configure Target"=w266:bool)  [unwired: 3 in]
        n166 = Current VI's Menubar() -> (w272:refnum<k9>)
        n167 = Set Menu Item Info(7:"Configure Target" ("item tag"), 8:w268, 9:w266, 11:w272) -> (0:w274:errorcluster, 3:w276:refnum<k9>)  [unwired: 3 out]
        n168 = Select(t=w257, s=w266, f=w256) -> (s? t:f=w265:T24)
        n169 = Select(t=w257, s=w264, f=w256) -> (s? t:f=w263:T24)
        n170 = Select(t=w257, s=w262, f=w256) -> (s? t:f=w261:T24)
        n171 = Select(t=w257, s=w260, f=w256) -> (s? t:f=w259:T24)
        n172 = Select(t=w257, s=w258, f=w256) -> (s? t:f=w255:T24)
        n173 = Set Menu Item Info(7:"Configure App Image" ("item tag"), 8:w274, 9:w264, 11:w276) -> (0:w277:errorcluster, 3:w278:refnum<k9>)  [unwired: 3 out]
        n174 = Set Menu Item Info(7:"View Target Info" ("item tag"), 8:w277, 9:w267, 11:w278) -> (0:w279:errorcluster, 3:w280:refnum<k9>)  [unwired: 3 out]
        n175 = Set Menu Item Info(7:"Deploy AppImage" ("item tag"), 8:w279, 9:w262, 11:w280) -> (0:w281:errorcluster, 3:w282:refnum<k9>)  [unwired: 3 out]
        n176 = property on="Property Node" class="Bool"("Disabled"=w265) -> ()  [unwired: 2 in, 2 out]
        n177 = property on="Property Node" class="Bool"("Disabled"=w263) -> ()  [unwired: 2 in, 2 out]
        n178 = property on="Property Node" class="Bool"("Disabled"=w261) -> ()  [unwired: 2 in, 2 out]
        n179 = property on="Property Node" class="Bool"("Disabled"=w259) -> ()  [unwired: 2 in, 2 out]
        n180 = property on="Property Node" class="Bool"("DisabledEnum"=w255) -> ()  [unwired: 2 in, 2 out]
        n181 = Set Menu Item Info(7:"Retrieve AppImage" ("item tag"), 8:w281, 9:w260, 11:w282) -> (0:w253:errorcluster, 3:w254:refnum<k9>)  [unwired: 3 out]
        n182 = Set Menu Item Info(7:"Convert Images" ("item tag"), 8:w253, 9:w250, 11:w254) -> (0:w252:errorcluster)  [unwired: 4 out]
      }
      frame "Status" {
      }
      frame "About" {
        # "Show About dialog"
        n183 = call "rad_About Dialog.vi"() -> ()  [unwired: 12 out]
      }
      frame "Error" {
        # "Display run-time error message\nAdd code to log error if desired"
        n184 = disable-structure shown="TARGET_TYPE==Windows" {
          disable-tunnel: w291 -> [w293 _]
          frame condition #0 (active) {
            n185 = call <vilib>:"Simple Error Handler.vi"("error in (no error)"=w293) -> ()  [unwired: 1 in, 8 out]
          }
          frame condition #1 {
          }
        }
      }
      frame "Exit" {
        # "Store current settings in the application config file"
        # "Close the front panel if the application is running as an EXE"
        n186 = Release Queue(queue=w305, force destroy? (F)=TRUE, error in (no error)=w304) -> (error out=w297:errorcluster)  [unwired: 2 out]
        n187 = Open Application Reference() -> (0:w302:errorcluster, 3:w303:refnum<vi>)  [unwired: 4 in]
        n188 = call "rad_Save Config.vi"("error in (no error"=w297, "State"=w298) -> ("error out"=w296:errorcluster)  [unwired: 1 in, 8 out]
        n189 = property class="App"(reference=w303, error in=w302) -> ("App.Kind"=w301:T25)  [unwired: 2 out]
        n190 = case shown="\"Run Time System\"" w301 {
          frame Default {
          }
          frame "Run Time System" {
            # "Close FP in EXE"
            n191 = Current VI's Path() -> (path=w308:path)
            n192 = Open VI Reference(vi path=w308) -> (vi reference=w307:refnum<vi>, error out=w306:errorcluster)  [unwired: 5 in]
            n193 = invoke class="VI" method="FP.Close"(reference=w307, error in=w306) -> ()  [unwired: 1 in, 3 out]
          }
        }
        n194 = property on="Property Node" class="Bool (strict)"(error in=w296, "Val(Sgnl)"=TRUE) -> (error out=w299:errorcluster)  [unwired: 1 in, 1 out]
      }
      frame "**** Target Messages ****" {
      }
      frame "Configure Discovery" {
        # "Refresh targets if:\n-It is the first iteration OR\n-Discovery settings were just changed"
        # "We ask the user to select the discovery \nmethod only if:\n-It is being called from the top\nmenu (not first) OR\n-The NotAsk flag hasn't been set to \nTrue (still ask me) in a first call"
        n195 = Unbundle By Name(w316) -> ("Discovery.NotAsk"=w315:bool)
        n196 = Equal?(x=w313, y="First") -> (x = y?=w311:bool)
        n197 = Compound Arithmetic op=OR(invert w315, invert w311) -> (w314:bool)
        n198 = case shown="True" w314 {
          tunnel: w316 -> [w329 w332]
          tunnel: [w329 w331] -> w322
          tunnel: [FALSE ("Changes?") w330] -> w317
          frame False {
          }
          frame True {
            # "This VI will ask the user\nhow to discover targets\non the network"
            n199 = call "rad_Configure Discovery Settings Dialog.vi"("Discovery Settings"=w332) -> ("Changes?"=w330:bool, "Discovery Settings out"=w331:T1)  [unwired: 9 in]
          }
        }
        n200 = Or(x=w317, y=w311) -> (x .or. y?=w318:bool)
        n201 = case shown="False" w318 {
          tunnel: [w323 w326] -> w321
          tunnel: w320 -> [_ w325]
          tunnel: w319 -> [w323 w324]
          frame False {
          }
          frame True {
            n202 = call "Enqueue Message with Data.vi"("error in (no error)"=w324, "message ID"="Refresh Targets" ("Message Name"), "queue in"=w325) -> ("error out"=w326:errorcluster)  [unwired: 7 in, 1 out]
          }
        }
      }
      frame "Refresh Targets" {
        # "Refresh list of RT targets on the local subnet.\nShow progress dialog during this process."
        n203 = Unbundle By Name(w341) -> ("Targets Settings.Reduce Discovery Timeout"=w334:bool, "User Added Targets"=w347:string[], "Targets Settings.Target Types"=w333:string[])
        n204 = call "Util_Progress Show Progress Popup.vi"("error in (no error)"=w337, "Title"="Discovering Targets", "Message"="Refreshing target list...") -> ("error out"=w335:errorcluster)  [unwired: 1 in, 7 out]
        n205 = Search 1D Array(1D array=w333, element="User Targets Only") -> (index of element=w344:i32)  [unwired: 1 in]
        n206 = Not Equal?(x=w344, y=-1) -> (x != y?=w342:bool)
        n207 = call "rad_Refresh Target Information.vi"("Reduce Discovery Timeout"=w334, "error in (no error)"=w335, "User Added Targets Only"=w342, "User Added Targets"=w347) -> ("error out"=w336:errorcluster, "Targets Information"=w346:T3[])  [unwired: 6 in]
        n208 = call "Util_Progress Close Progress Popup.vi"("error in (no error)"=w336) -> ()  [unwired: 2 in, 9 out]
        n209 = Bundle By Name(cluster=w341, "Targets Information"=w346) -> (w340:T1)
        n210 = call "Enqueue Message with Data.vi"("error in (no error)"=w336, "message ID"="Update UI", "queue in"=w338) -> ("error out"=w339:errorcluster)  [unwired: 7 in, 1 out]
      }
      frame "Add Target to List" {
        n211 = Unbundle By Name(w357) -> ("User Added Targets"=w359:string[])
        n212 = call "rad_Add Target By IP Dialog.vi"() -> ("Canceled?"=w351:bool, "IP Address"=w358:string)  [unwired: 10 in]
        n213 = case shown="False" w351 {
          tunnel: w359 -> [w367 w372]
          tunnel: w358 -> [w366 _]
          tunnel: [w368 w372] -> w355
          frame False {
            n214 = Search 1D Array(1D array=w367, element=w366) -> (index of element=w371:i32)  [unwired: 1 in]
            n215 = Build Array (concatenate)(w367, w366) -> (w365:string[])
            n216 = Not Equal?(x=w371, y=-1) -> (x != y?=w369:bool)
            n217 = Select(t=w367, s=w369, f=w365) -> (s? t:f=w368:string[])
          }
          frame True {
          }
        }
        n218 = case shown="False" w351 {
          tunnel: w354 -> [w363 w364]
          tunnel: [w362 w364] -> w353
          tunnel: w352 -> [w361 _]
          frame False {
            n219 = call "Enqueue Message with Data.vi"("error in (no error)"=w363, "message ID"="Refresh Targets" ("Message Name"), "queue in"=w361) -> ("error out"=w362:errorcluster)  [unwired: 7 in, 1 out]
          }
          frame True {
          }
        }
        n220 = Bundle By Name(cluster=w357, "User Added Targets"=w355) -> (w356:T1)
      }
      frame "Configure Target" {
        # "Update network settings/configuration of the selected RT target"
        n221 = Unbundle By Name(w379) -> ("Targets Information"=w383:T3[], "Filtered Targets"=w386:i32[])
        n222 = Decimal String To Number(string=w387) -> (number=w385:i32)  [unwired: 3 out]
        n223 = Index Array(array=w386, index=w385) -> (element=w381:i32)
        n224 = Index Array(array=w383, index=w381) -> (element=w384:T3)
        n225 = call "rad_Configure Target Dialog.vi"("Error In"=w373, "Target Information in"=w384) -> ("Error Out"=w374:errorcluster, "Target Information out"=w382:T3)  [unwired: 8 out]
        n226 = Replace Array Subset(array=w383, new element=w382, index=w381) -> (w380:T3[])
        n227 = call <vilib>:"General Error Handler.vi"("error in (no error)"=w374) -> ()  [unwired: 10 in, 5 out]
        n228 = Bundle By Name(cluster=w379, "Targets Information"=w380) -> (w378:T1)
        n229 = call "Enqueue Message with Data.vi"("error in (no error)"=w373, "message ID"="Update UI", "queue in"=w377) -> ("error out"=w375:errorcluster)  [unwired: 7 in, 1 out]
      }
      frame "Configure Targets Settings" {
        # "Update the RT Target settings >> select which types of RT targets to display in the table\nCompactRIO, PXI, FieldPoint, or Other"
        n230 = Unbundle By Name(w395) -> ("Targets Settings"=w390:T2)
        n231 = call "rad_Configure Targets Settings Dialog.vi"("Targets Settings"=w390) -> ("Targets Settings"=w391:T2)  [unwired: 10 out]
        n232 = Equal?(x=w391, y=w390) -> (x = y?=w388:bool)
        n233 = Bundle By Name(cluster=w395, "Targets Settings"=w391) -> (w394:T1)
        n234 = case shown="False" w388 {
          tunnel: w393 -> [w399 _]
          tunnel: w392 -> [w398 w400]
          tunnel: [w397 w400] -> w389
          frame False {
            n235 = call "Enqueue Message with Data.vi"("error in (no error)"=w398, "message ID"="Update UI", "queue in"=w399) -> ("error out"=w397:errorcluster)  [unwired: 7 in, 1 out]
          }
          frame True {
          }
        }
      }
      frame "View Target Info" {
        # "Display additional information about the selected RT target in a popup window"
        n236 = Unbundle By Name(w410) -> ("Targets Information"=w409:T3[], "Filtered Targets"=w407:i32[])
        n237 = Decimal String To Number(string=w408) -> (number=w406:i32)  [unwired: 3 out]
        n238 = Index Array(array=w407, index=w406) -> (element=w405:i32)
        n239 = Index Array(array=w409, index=w405) -> (element=w401:T3)
        n240 = call "rad_Get Target Info (IP).vi"("error in (no error)"=w403, "Target settings in"=w401) -> ("error out"=w402:errorcluster, "Target settings out"=w404:T3)  [unwired: 8 in]
        n241 = case shown="No Error" w402 {
          selector: w402 -> [_ w412]
          tunnel: w404 -> [w411 _]
          frame No Error {
            n242 = call "rad_Target Info Dialog.vi"("Target Information"=w411) -> ()  [unwired: 11 out]
          }
          frame Error {
            n243 = call <vilib>:"General Error Handler.vi"("error in (no error)"=w412) -> ()  [unwired: 10 in, 5 out]
          }
        }
      }
      frame "Delete Target" {
        n244 = Unbundle By Name(w428) -> ("Targets Information"=w427:T3[], "Filtered Targets"=w415:i32[], "User Added Targets"=w416:string[])
        n245 = Decimal String To Number(string=w432) -> (number=w418:i32)  [unwired: 2 in, 1 out]
        n246 = Index Array(array=w415, index=w418) -> (element=w417:i32)
        n247 = Delete From Array(array=w427, length=1, index=w417) -> (deleted portion=w425:T3[], array with subset deleted=w426:T3[])
        n248 = Index Array(array=w425) -> (element=w424:T3)  [unwired: 1 in]
        n249 = Unbundle By Name(w424) -> ("Primary NIC.IP address"=w414:string)
        n250 = Search 1D Array(1D array=w416, element=w414) -> (index of element=w431:i32)  [unwired: 1 in]
        n251 = call "Enqueue Message with Data.vi"("error in (no error)"=w421, "message ID"="Update UI" ("Message Name"), "queue in"=w422) -> ("error out"=w420:errorcluster)  [unwired: 7 in, 1 out]
        n252 = Delete From Array(array=w416, length=1, index=w431) -> (array with subset deleted=w413:string[])  [unwired: 1 out]
        n253 = Bundle By Name(cluster=w428, "Targets Information"=w426, "User Added Targets"=w413) -> (w423:T1)
      }
      frame "**** Image Messages ****" {
      }
      frame "Refresh AppImages" {
        # "Update list of application images available in the configured folder"
        n254 = Unbundle By Name(w440) -> ("App Images Settings.App Images Temp Folder"=w441:path, "App Images Settings.App Images Folder"=w445:path)
        n255 = call "Util_Progress Show Progress Popup.vi"("Title"="Refreshing App Images", "Message"="Refreshing application images list...") -> ("error out"=w444:errorcluster)  [unwired: 2 in, 7 out]
        n256 = call "rad_List Application Images.vi"("App Image Temp Folder"=w441, "error in (no error)"=w444, "App Images Folder"=w445) -> ("error out"=w443:errorcluster, "Application Images Infomration"=w442:T6[])  [unwired: 1 in, 6 out]
        n257 = Bundle By Name(cluster=w440, "App Images Information"=w442) -> (w436:T1)
        n258 = call "Util_Progress Close Progress Popup.vi"("error in (no error)"=w443) -> ()  [unwired: 2 in, 9 out]
        n259 = call "Enqueue Message with Data.vi"("error in (no error)"=w437, "message ID"="Update UI" ("Message"), "queue in"=w438) -> ("error out"=w439:errorcluster)  [unwired: 7 in, 1 out]
      }
      frame "Configure App Image" {
        # "Update additional information (name, verison, description)\nstored with the selected application image"
        n260 = Unbundle By Name(w458) -> ("App Images Settings.App Images Temp Folder"=w454:path, "App Images Information"=w460:T6[])
        n261 = Decimal String To Number(string=w461) -> (number=w456:i32)  [unwired: 3 out]
        n262 = Index Array(array=w460, index=w456) -> (element=w455:T6)
        n263 = call "rad_Configure Application Image.vi"("Temp Folder"=w454, "error in (no error)"=w453, "App Images Information"=w455) -> ("error out"=w450:errorcluster, "Cancelled"=w448:bool, "App Images Information"=w449:T6)  [unwired: 6 in]
        n264 = Replace Array Subset(array=w460, new element=w449, index=w456) -> (w459:T6[])
        n265 = case shown="False" w448 {
          tunnel: [w465 w466] -> w452
          tunnel: w451 -> [w463 _]
          tunnel: w450 -> [w462 w466]
          frame False {
            n266 = call "Enqueue Message with Data.vi"("error in (no error)"=w462, "message ID"="Refresh AppImages", "queue in"=w463) -> ("error out"=w465:errorcluster)  [unwired: 7 in, 1 out]
          }
          frame True {
          }
        }
        n267 = Bundle By Name(cluster=w458, "App Images Information"=w459) -> (w457:T1)
      }
      frame "Configure AppImages Settings" {
        # "Update the selection of the folder where application images are stored"
        n268 = Unbundle By Name(w471) -> ("App Images Settings"=w470:T5)
        n269 = call "rad_Configure App Images Settings Dialog.vi"("App Images Settings"=w470) -> ("Cancelled"=w467:bool, "App Images Settings"=w469:T5)  [unwired: 1 in, 8 out]
        n270 = case shown="False" w467 {
          tunnel: w474 -> [w478 _]
          tunnel: w473 -> [w476 w479]
          tunnel: [w475 w479] -> w468
          frame False {
            n271 = call "Enqueue Message with Data.vi"("error in (no error)"=w476, "message ID"="Refresh AppImages", "queue in"=w478) -> ("error out"=w475:errorcluster)  [unwired: 7 in, 1 out]
          }
          frame True {
          }
        }
        n272 = Bundle By Name(cluster=w471, "App Images Settings"=w469) -> (w472:T1)
      }
      frame "View App Image Info" {
        n273 = Unbundle By Name(w484) -> ("App Images Information"=w483:T6[])
        n274 = Decimal String To Number(string=w481) -> (number=w480:i32)  [unwired: 2 in, 1 out]
        n275 = Index Array(array=w483, index=w480) -> (element=w482:T6)
        n276 = call "rad_View App Image Info.vi"("App Images Information"=w482) -> ()  [unwired: 11 in]
      }
      frame "Compare App Image" {
        n277 = Scan From String(format string="%[^(]", input string=w488) -> (remaining string=w487:string, output 1=w489:string)  [unwired: 2 in, 3 out]
        n278 = case shown="\"Image Target Compare\"" w489 {
          tunnel: w492 -> [w504 w533 w539]
          tunnel: w491 -> [w501 w525 w544]
          tunnel: w487 -> [w503 w535 _]
          tunnel: [w496 w523 w543] -> w486
          frame "Image Target Compare" {
            n279 = Unbundle By Name(w504) -> ("App Images Settings.App Images Folder"=w495:path, "App Images Settings.App Images Temp Folder"=w499:path, "App Images Information"=w509:T6[], "Targets Information"=w505:T3[], "Filtered Targets"=w506:i32[])
            n280 = Scan From String(format string="(%[^)]):%d", input string=w503, error in=w501) -> (error out=w497:errorcluster, output 1=w508:string, output 2=w510:i32)  [unwired: 1 in, 4 out]
            n281 = while {
              shift-right: [w518] -> _
              shift-left: w508 -> [w520]
              tunnel: w506 -> [w515]
              tunnel: w505 -> [w513]
              tunnel: [w512] -> w502 mode=indexing
              stop <- w517 stop-if-true
              n282 = Scan From String(format string="%d,", input string=w520) -> (remaining string=w518:string, output 1=w514:i32)  [unwired: 2 in, 3 out]
              n283 = Index Array(array=w515, index=w514) -> (element=w516:i32)
              n284 = Empty String/Path?(string/path=w518) -> (empty?=w517:bool)
              n285 = Index Array(array=w513, index=w516) -> (element=w512:T3)
            }
            n286 = Index Array(array=w509, index=w510) -> (element=w507:T6)
            n287 = Index Array(array=w502) -> (element=w493:T3)  [unwired: 1 in]
            n288 = Unbundle By Name(w507) -> ("AppImage Path"=w500:path)
            n289 = call "rad_RT Image Compare Dialog.vi"("App Images Repository"=w495, "Begin Automatically? (F)"=TRUE ("Show Front Panel?"), "Temp Folder"=w499, "error in (no error)"=w497, "Operation"=rad_Comparison_Modes."Compare Local Image With Controller", "Target settings"=w493, "Original Image Path"=w500) -> ("error out"=w496:errorcluster)  [unwired: 4 in]
          }
          frame "Only Image Selected" {
            n290 = Unbundle By Name(w533) -> ("App Images Settings.App Images Folder"=w522:path, "App Images Settings.App Images Temp Folder"=w528:path, "App Images Information"=w532:T6[])
            n291 = Scan From String(format string="(%d", input string=w535, error in=w525) -> (error out=w524:errorcluster, output 1=w531:i32)  [unwired: 1 in, 3 out]
            n292 = Index Array(array=w532, index=w531) -> (element=w530:T6)
            n293 = Unbundle By Name(w530) -> ("AppImage Path"=w529:path)
            n294 = call "rad_RT Image Compare Dialog.vi"("App Images Repository"=w522, "Begin Automatically? (F)"=FALSE ("Operate Headlessly?"), "Temp Folder"=w528, "error in (no error)"=w524, "Operation"=rad_Comparison_Modes."Compare Local Image With Controller", "Target settings"=T3 {"Hostname"="", "Serial number"="", "Product name"="", "Product code"=0, "System status"="", "Credential type"=enum."None/Unlocked", "User added?"=FALSE, "Primary NIC"={"MAC address"="", "IP Address Request Mode"=0, "IP address"="", "Subnet mask"="", "Gateway"="", "DNS server"=""}}, "Original Image Path"=w529) -> ("error out"=w523:errorcluster)  [unwired: 4 in]
          }
          frame "Generic Compare", Default {
            n295 = Unbundle By Name(w539) -> ("App Images Settings.App Images Folder"=w537:path, "App Images Settings.App Images Temp Folder"=w538:path)
            n296 = call "rad_RT Image Compare Dialog.vi"("App Images Repository"=w537, "Begin Automatically? (F)"=FALSE ("Operate Headlessly?"), "Temp Folder"=w538, "error in (no error)"=w544, "Operation"=rad_Comparison_Modes."Compare Local Image With Controller", "Target settings"=T3 {"Hostname"="", "Serial number"="", "Product name"="", "Product code"=0, "System status"="", "Credential type"=enum."None/Unlocked", "User added?"=FALSE, "Primary NIC"={"MAC address"="", "IP Address Request Mode"=0, "IP address"="", "Subnet mask"="", "Gateway"="", "DNS server"=""}}, "Original Image Path"=path "") -> ("error out"=w543:errorcluster)  [unwired: 4 in]
          }
        }
      }
      frame "Delete App Image" {
        n297 = Unbundle By Name(w561) -> ("App Images Information"=w560:T6[])
        n298 = Decimal String To Number(string=w559) -> (number=w558:i32)  [unwired: 2 in, 1 out]
        n299 = Index Array(array=w560, index=w558) -> (element=w557:T6)
        n300 = Unbundle By Name(w557) -> ("AppImage Path"=w552:path, "AppImage Properties.Name"=w554:string, "AppImage Properties.Version"=w545:string)
        n301 = Concatenate Strings("Are you sure you want to delete " ("string"), w554, " version " ("string"), w545, "?" ("string")) -> (w553:string)
        n302 = Two Button Dialog(message=w553, 2:"Delete" ("button name (\"OK\")")) -> (T button?=w551:bool)  [unwired: 1 in]
        n303 = case shown="True" w551 {
          tunnel: w552 -> [_ w568]
          tunnel: w550 -> [w562 w567]
          tunnel: [w562 w565] -> w549
          tunnel: w548 -> [_ w564]
          frame False {
          }
          frame True {
            n304 = Delete(path (use dialog)=w568, error in=w567) -> (error out=w566:errorcluster)  [unwired: 3 in, 2 out]
            n305 = call "Enqueue Message with Data.vi"("error in (no error)"=w566, "message ID"="Refresh AppImages" ("Message Name"), "queue in"=w564) -> ("error out"=w565:errorcluster)  [unwired: 7 in, 1 out]
          }
        }
      }
      frame "Retrieve AppImage" {
        # "Retrieve the application image\nfrom the selected RT target."
        n306 = Unbundle By Name(w577) -> ("App Images Settings.App Images Temp Folder"=w579:path, "App Images Settings.App Images Folder"=w573:path, "Targets Information"=w569:T3[], "Filtered Targets"=w570:i32[])
        n307 = Decimal String To Number(string=w585) -> (number=w584:i32)  [unwired: 3 out]
        n308 = Index Array(array=w570, index=w584) -> (element=w586:i32)
        n309 = Index Array(array=w569, index=w586) -> (element=w571:T3)
        n310 = call "rad_Retrieve Application Image From Target.vi"("App Images Temp Folder"=w579, "error in (no error)"=w583, "Target settings"=w571, "App Images Folder"=w573) -> ("error out"=w582:errorcluster, "Cancelled"=w574:bool, "New App Image Path"=w578:path)  [unwired: 3 in, 2 out]
        n311 = Strip Path(path=w578) -> (stripped path=w575:path)  [unwired: 1 out]
        n312 = case shown="False" w574 {
          tunnel: w582 -> [w590 w591]
          tunnel: [w589 w591] -> w581
          tunnel: w580 -> [w588 _]
          frame False {
            n313 = call "Enqueue Message with Data.vi"("error in (no error)"=w590, "message ID"="Refresh AppImages" ("Message Name"), "queue in"=w588) -> ("error out"=w589:errorcluster)  [unwired: 7 in, 1 out]
          }
          frame True {
          }
        }
        n314 = Select(t=w573, s=w574, f=w575) -> (s? t:f=w572:path)
        n315 = Bundle By Name(cluster=w577, "App Images Settings.App Images Folder"=w572) -> (w576:T1)
      }
      frame "Deploy AppImage" {
        # "Deploy the selected application image to the select RT target(s)"
        n316 = Unbundle By Name(w608) -> ("App Images Settings.App Images Temp Folder"=w598:path, "App Images Information"=w604:T6[], "Targets Information"=w600:T3[], "Filtered Targets"=w601:i32[])
        n317 = Scan From String(format string="(%[^)]):%d", input string=w607) -> (output 1=w603:string, output 2=w605:i32)  [unwired: 2 in, 5 out]
        n318 = while {
          shift-right: [w620] -> _
          shift-left: w603 -> [w622]
          tunnel: w601 -> [w617]
          tunnel: w600 -> [w615]
          tunnel: [w614] -> w597 mode=indexing
          stop <- w619 stop-if-true
          n319 = Scan From String(format string="%d,", input string=w622) -> (remaining string=w620:string, output 1=w616:i32)  [unwired: 2 in, 3 out]
          n320 = Index Array(array=w617, index=w616) -> (element=w618:i32)
          n321 = Empty String/Path?(string/path=w620) -> (empty?=w619:bool)
          n322 = Index Array(array=w615, index=w618) -> (element=w614:T3)
        }
        n323 = Index Array(array=w604, index=w605) -> (element=w602:T6)
        n324 = Unbundle By Name(w602) -> ("AppImage Path"=w599:path)
        n325 = call "rad_Deploy Application Image.vi"("App Image Temp Folder"=w598, "error in (no error)"=w596, "Selected Targets"=w597, "App Image Path"=w599) -> ("error out"=w594:errorcluster, "Cancelled"=w592:bool)  [unwired: 6 out]
        n326 = case shown="False" w592 {
          tunnel: [w612 w613] -> w595
          tunnel: w594 -> [w611 w613]
          tunnel: w593 -> [w609 _]
          frame False {
            n327 = call "Enqueue Message with Data.vi"("error in (no error)"=w611, "message ID"="Refresh Targets" ("Message Name"), "queue in"=w609) -> ("error out"=w612:errorcluster)  [unwired: 7 in, 1 out]
          }
          frame True {
          }
        }
      }
      frame "Convert Images" {
        n328 = Unbundle By Name(w624) -> ("App Images Settings.App Images Folder"=w623:path)
        n329 = call "Util_ConvertImageToLatest.vi"("error in (no error)"=w629, "Image Path"=w623) -> ("error out"=w627:errorcluster)  [unwired: 9 in]
        n330 = call "Enqueue Message with Data.vi"("error in (no error)"=w627, "message ID"="Refresh AppImages" ("Message Name"), "queue in"=w625) -> ("error out"=w626:errorcluster)  [unwired: 7 in, 1 out]
      }
    }
    n331 = local write item#-1(w145) -> ()
  }
